vi "Init Tx - Conversion Resources.vi"(8 "error in (no error)":errorcluster, 11 "Tx Loop Data":T1) -> (0 "error out":errorcluster, 3 "Tx Loop Data out":T1)   [LabVIEW 2016, in "UDP-Custom-Device Engine.lvlib"]
uses:
  UDP-Custom-Device Engine.lvlib
  Types/Engine - Tx Loop Data.ctl
  <vilib>/NI Veristand/VeriStand Data/Byte Buffer/Byte Buffer.lvclass
  Types/Engine - General Resources.ctl
  <vilib>/NI Veristand/VeriStand Data/Typedefs/Typedefs.Data Types.ctl
  Shared/Types/Shared - Duplex Settings.ctl
  Shared/Types/Shared - Header Details.ctl
  Types/Engine - Data Conversion Config.ctl
  <vilib>/NI Veristand/VeriStand Data/Byte Buffer/Byte Buffer.Mapping.ctl
  Types/Engine - Tx Runtime Resources.ctl
  Shared/Types/Shared - Transmit Flag Options.ctl
  Types/Engine - Tx Echo Resources.ctl
  Shared/Types/Shared - Transmit Echo Options.ctl
  Types/Engine - Tx Channel Refs.ctl
  <vilib>/NI/NIVS Inline Async API/_Data Access Engine/Data Access Engine/Types/Read.DVR.ctl
  <vilib>/NI/NIVS Inline Async API/_Data Access Engine/Access Type Classes/Read/Read.lvclass
  <vilib>/NI/NIVS Inline Async API/_Data Access Engine/Data Access Engine/Types/Write.DVR.ctl
  <vilib>/NI/NIVS Inline Async API/_Data Access Engine/Access Type Classes/Write/Write.lvclass
  Types/Engine - Debug Resources.ctl
  <vilib>/NI Veristand/VeriStand Data/Byte Buffer/Byte Buffer.lvclass/Byte Buffer.ctl
  <vilib>/NI Veristand/VeriStand Data/Byte Buffer/Byte Buffer.Mapping.Create (Channel Pointer).vi
  <vilib>/NI Veristand/VeriStand Data/Utilities/Utilities.Sizeof.Array.vi
  <vilib>/NI Veristand/VeriStand Data/Memory Management/Memory Management.MoveDblBlock.Write (Double).vi
  <vilib>/NI Veristand/VeriStand Data/Byte Buffer/Byte Buffer.Write.Typed Double Array.vi
  <vilib>/NI Veristand/VeriStand Data/Utilities/Utilities.Buffer.Double.vi
  <vilib>/NI Veristand/VeriStand Data/Utilities/Utilities.Sizeof.Scalar.vi
  <vilib>/NI Veristand/VeriStand Data/Byte Buffer/Byte Buffer.Write.vi
  <vilib>/NI Veristand/VeriStand Data/Byte Buffer/Byte Buffer.Write (1D Boolean).vi
  <vilib>/NI Veristand/VeriStand Data/Type Conversion/Type Conversion.From Double.Subset.vi
  <vilib>/NI Veristand/VeriStand Data/Type Conversion/Type Conversion.From Double.Subset (1D Boolean).vi
  <vilib>/NI Veristand/VeriStand Data/Byte Buffer/Byte Buffer.Write (1D SGL).vi
  <vilib>/NI Veristand/VeriStand Data/Type Conversion/Type Conversion.From Double.Subset (1D SGL).vi
  <vilib>/NI Veristand/VeriStand Data/Byte Buffer/Byte Buffer.Write (1D DBL).vi
  <vilib>/NI Veristand/VeriStand Data/Byte Buffer/Byte Buffer.Write (1D I8).vi
  <vilib>/NI Veristand/VeriStand Data/Type Conversion/Type Conversion.From Double.Subset (1D I8).vi
  <vilib>/NI Veristand/VeriStand Data/Byte Buffer/Byte Buffer.Write (1D I16).vi
  <vilib>/NI Veristand/VeriStand Data/Type Conversion/Type Conversion.From Double.Subset (1D I16).vi
  <vilib>/NI Veristand/VeriStand Data/Byte Buffer/Byte Buffer.Write (1D I32).vi
  <vilib>/NI Veristand/VeriStand Data/Type Conversion/Type Conversion.From Double.Subset (1D I32).vi
  <vilib>/NI Veristand/VeriStand Data/Byte Buffer/Byte Buffer.Write (1D I64).vi
  <vilib>/NI Veristand/VeriStand Data/Type Conversion/Type Conversion.From Double.Subset (1D I64).vi
  <vilib>/NI Veristand/VeriStand Data/Byte Buffer/Byte Buffer.Write (1D U8).vi
  <vilib>/NI Veristand/VeriStand Data/Type Conversion/Type Conversion.From Double.Subset (1D U8).vi
  <vilib>/NI Veristand/VeriStand Data/Byte Buffer/Byte Buffer.Write (1D U16).vi
  <vilib>/NI Veristand/VeriStand Data/Type Conversion/Type Conversion.From Double.Subset (1D U16).vi
  <vilib>/NI Veristand/VeriStand Data/Byte Buffer/Byte Buffer.Write (1D U32).vi
  <vilib>/NI Veristand/VeriStand Data/Type Conversion/Type Conversion.From Double.Subset (1D U32).vi
  <vilib>/NI Veristand/VeriStand Data/Byte Buffer/Byte Buffer.Write (1D U64).vi
  <vilib>/NI Veristand/VeriStand Data/Type Conversion/Type Conversion.From Double.Subset (1D U64).vi
  <vilib>/NI Veristand/VeriStand Data/Byte Buffer/Byte Buffer.Write (String).vi
  <vilib>/NI Veristand/VeriStand Data/Type Conversion/Type Conversion.From Double.vi
  <vilib>/NI Veristand/VeriStand Data/Type Conversion/Type Conversion.From Double (1D Boolean).vi
  <vilib>/NI Veristand/VeriStand Data/Type Conversion/Type Conversion.From Double (1D SGL).vi
  <vilib>/NI Veristand/VeriStand Data/Type Conversion/Type Conversion.From Double (1D I8).vi
  <vilib>/NI Veristand/VeriStand Data/Type Conversion/Type Conversion.From Double (1D I16).vi
  <vilib>/NI Veristand/VeriStand Data/Type Conversion/Type Conversion.From Double (1D I32).vi
  <vilib>/NI Veristand/VeriStand Data/Type Conversion/Type Conversion.From Double (1D I64).vi
  <vilib>/NI Veristand/VeriStand Data/Type Conversion/Type Conversion.From Double (1D U8).vi
  <vilib>/NI Veristand/VeriStand Data/Type Conversion/Type Conversion.From Double (1D U16).vi
  <vilib>/NI Veristand/VeriStand Data/Type Conversion/Type Conversion.From Double (1D U32).vi
  <vilib>/NI Veristand/VeriStand Data/Type Conversion/Type Conversion.From Double (1D U64).vi
  <vilib>/NI Veristand/VeriStand Data/Byte Buffer/Byte Buffer.Subset.Set.vi
  <vilib>/NI Veristand/VeriStand Data/Byte Buffer/Byte Buffer.Get Buffer Pointer.vi
  <vilib>/NI Veristand/VeriStand Data/Byte Buffer/Byte Buffer.Get Buffer Size.vi
  <vilib>/NI Veristand/VeriStand Data/Memory Management/Memory Management.MoveByteBlock.Read (String).vi
  <vilib>/NI Veristand/VeriStand Data/Memory Management/Memory Management.Handle Return.vi
  <vilib>/NI Veristand/VeriStand Data/Byte Buffer/Byte Buffer.Get Byte Order.vi
  <vilib>/NI Veristand/VeriStand Data/VeriStand Data.lvlib
  <vilib>/NI/NIVS Inline Async API/_Data Access Engine/Data Access Engine/Data Access Engine.lvclass
  Shared/UDP-Custom-Device Shared.lvlib
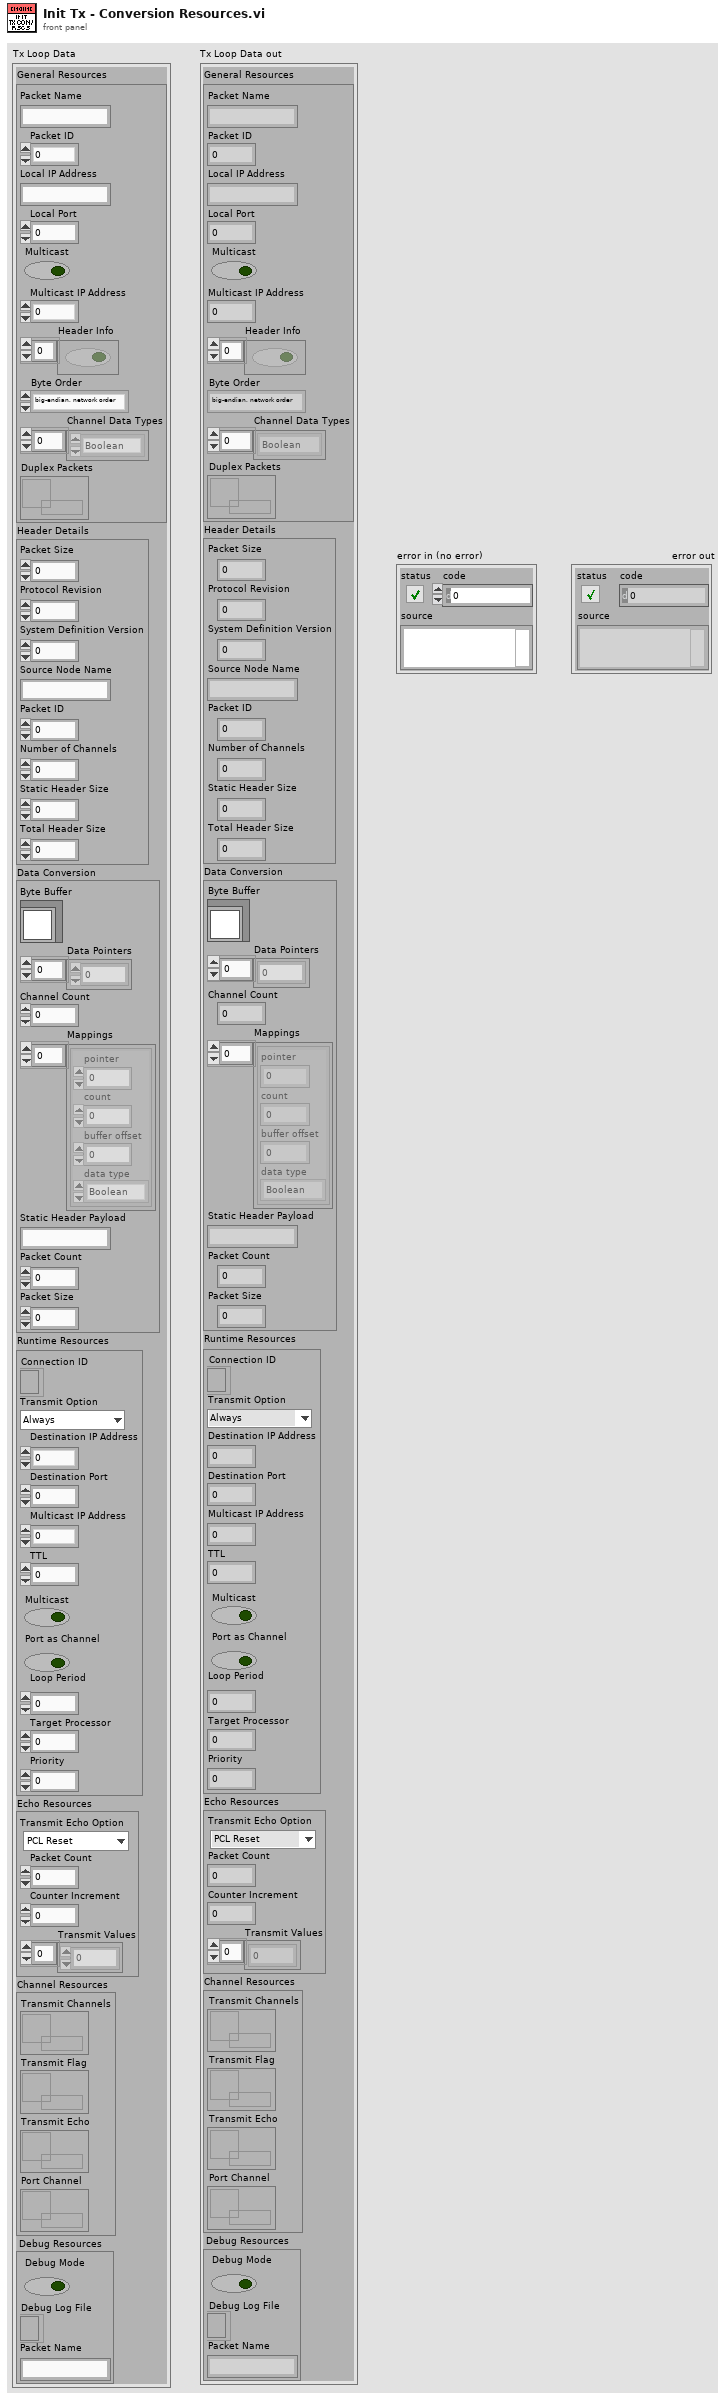
[diagram p1: front panel]
types:
  T1 = typedef "UDP-Custom-Device Engine.lvlib/Engine - Tx Loop Data.ctl" = cluster{"General Resources":T2, "Header Details":T4, "Data Conversion":T5, "Runtime Resources":T7, "Echo Resources":T9, "Channel Resources":T11, "Debug Resources":T14}
  T2 = typedef "UDP-Custom-Device Engine.lvlib/Engine - General Resources.ctl" = cluster{"Packet Name":string, "Packet ID":i32, "Local IP Address":string, "Local Port":i32, "Multicast":bool, "Multicast IP Address":u32, "Header Info":bool[], "Byte Order":enum16{"big-endian, network order", "native, host order", "little-endian"}, "Channel Data Types":T3[], "Duplex Packets":refnum<data-value>}
  T3 = typedef "VeriStand Data.lvlib/Typedefs.Data Types.ctl" = enum16{"Boolean", "Single", "Double", "I8", "I16", "I32", "I64", "U8", "U16", "U32", "U64"}
  T4 = typedef "UDP-Custom-Device Shared.lvlib/Shared - Header Details.ctl" = cluster{"Packet Size":u16, "Protocol Revision":u8, "System Definition Version":u64, "Source Node Name":string, "Packet ID":u32, "Number of Channels":u32, "Static Header Size":u16, "Total Header Size":u16}
  T5 = typedef "UDP-Custom-Device Engine.lvlib/Engine - Data Conversion Config.ctl" = cluster{"Byte Buffer":refnum<class "Byte Buffer.lvclass">, "Data Pointers":u64[], "Channel Count":i32, "Mappings":T6[], "Static Header Payload":string, "Packet Count":dbl, "Packet Size":i32}
  T6 = typedef "VeriStand Data.lvlib/Byte Buffer.lvclass/Byte Buffer.Mapping.ctl" = cluster{"pointer":u64, "count":i64, "buffer offset":u64, "data type":T3}
  T7 = typedef "UDP-Custom-Device Engine.lvlib/Engine - Tx Runtime Resources.ctl" = cluster{"Connection ID":refnum<k16>, "Transmit Option":T8, "Destination IP Address":u32, "Destination Port":u16, "Multicast IP Address":u32, "TTL":u16, "Multicast":bool, "Port as Channel":bool, "Loop Period":u32, "Target Processor":i32, "Priority":i32}
  T8 = typedef "UDP-Custom-Device Shared.lvlib/Shared - Transmit Flag Options.ctl" = enum16{"Always", "One-Shot", "Toggle"}
  T9 = typedef "UDP-Custom-Device Engine.lvlib/Engine - Tx Echo Resources.ctl" = cluster{"Transmit Echo Option":T10, "Packet Count":dbl, "Counter Increment":dbl, "Transmit Values":dbl[]}
  T10 = typedef "UDP-Custom-Device Shared.lvlib/Shared - Transmit Echo Options.ctl" = enum16{"PCL Reset", "Counter", "Mirror"}
  T11 = typedef "UDP-Custom-Device Engine.lvlib/Engine - Tx Channel Refs.ctl" = cluster{"Transmit Channels":T12, "Transmit Flag":T12, "Transmit Echo":T13, "Port Channel":T12}
  T12 = typedef "Data Access Engine.lvlib/Data Access Engine.lvclass/Read.DVR.ctl" = refnum<data-value>
  T13 = typedef "Data Access Engine.lvlib/Data Access Engine.lvclass/Write.DVR.ctl" = refnum<data-value>
  T14 = typedef "UDP-Custom-Device Engine.lvlib/Engine - Debug Resources.ctl" = cluster{"Debug Mode":bool, "Debug Log File":refnum<file>, "Packet Name":string}
  T15 = enum16{"big-endian, network order", "native, host order", "little-endian"}
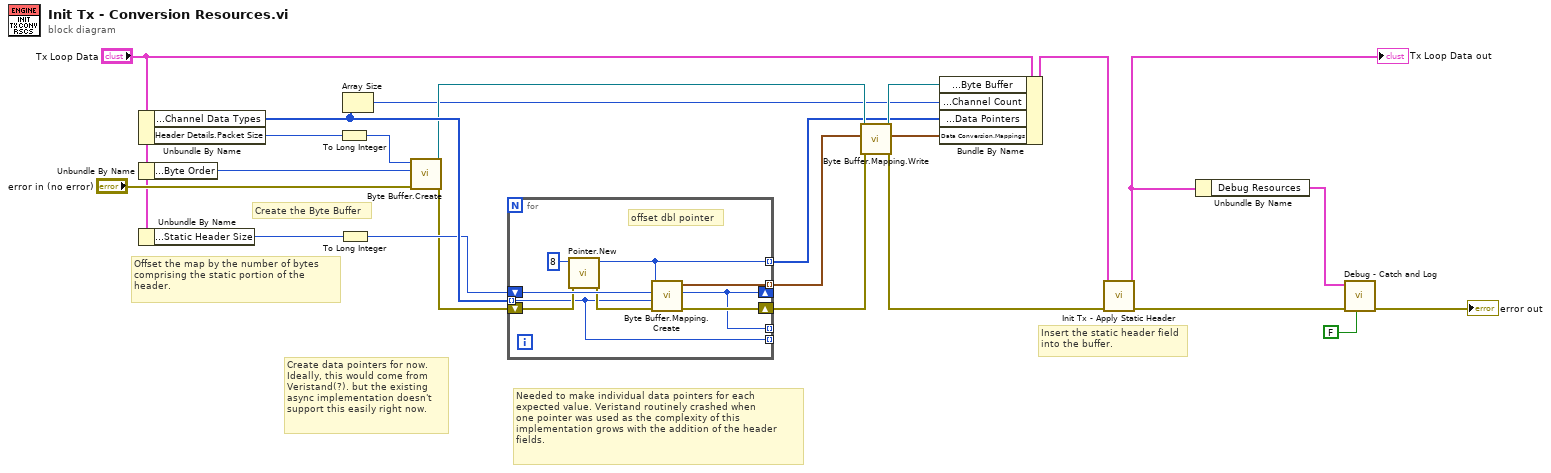
[diagram p0: block diagram]
diagram:
  # "Needed to make individual data pointers for each\nexpected value. Veristand routinely crashed when\none pointer was used as the complexity of this\nimplementation grows with the addition of the header\nfields."
  # "Insert the static header field\ninto the buffer."
  # "Offset the map by the number of bytes\ncomprising the static portion of the\nheader."
  # "Create the Byte Buffer"
  # "Create data pointers for now.\nIdeally, this would come from\nVeristand(?). but the existing\nasync implementation doesn't\nsupport this easily right now."
  n1 = Unbundle By Name("Tx Loop Data") -> ("General Resources.Channel Data Types"=w22:T3[], "Header Details.Packet Size"=w20:u16)
  n2 = Unbundle By Name("Tx Loop Data") -> ("General Resources.Byte Order"=w23:T15)
  n3 = Unbundle By Name("Tx Loop Data") -> ("Header Details.Static Header Size"=w17:u16)
  n4 = To Long Integer(number=w20) -> (32bit integer=w10:i32)
  n5 = To Long Integer(number=w17) -> (32bit integer=w9:i32)
  n6 = Array Size(array=w22) -> (size(s)=w8:i32)
  n7 = call <vilib>:"Byte Buffer.Create.vi"("error in (no error)"="error in (no error)", "byte order (big-endian)"=w23, "size"=w10) -> ("error out"=w7:errorcluster, "Byte Buffer"=w16:refnum<class "Byte Buffer.lvclass">)  [unwired: 7 in]
  n8 = for {
    tunnel: [w32] -> w13 mode=indexing
    tunnel: w22 -> [w24] mode=indexing
    shift-right: [w31] -> w12
    shift-left: w7 -> [w29]
    shift-right: [w25] -> _
    shift-left: w9 -> [w30]
    tunnel: [w26] -> w6 mode=indexing
    tunnel: [w25] -> _ mode=indexing
    tunnel: [w24] -> _ mode=indexing
    # "offset dbl pointer"
    n9 = call <vilib>:"Pointer.New.vi"("error in (no error)"=w29, "size in bytes"=8) -> ("error out"=w28:errorcluster, "pointer"=w26:u64)  [unwired: 8 in]
    n10 = call-poly <vilib>:"Byte Buffer.Mapping.Create.vi"("error in (no error)"=w28, "data type"=w24, "buffer offset"=w30, "Channel Pointer"=w26) -> ("error out"=w31:errorcluster, "new buffer offset"=w25:u64, "mapping"=w32:T6)  [unwired: 5 in]
  }
  n11 = call <vilib>:"Byte Buffer.Mapping.Write.vi"("error in (no error)"=w12, "mappings"=w13, "Byte Buffer in"=w16) -> ("error out"=w11:errorcluster, "mappings dup"=w14:T6[], "Byte Buffer out"=w15:refnum<class "Byte Buffer.lvclass">)  [unwired: 6 in]
  n12 = Bundle By Name(cluster="Tx Loop Data", "Data Conversion.Byte Buffer"=w15, "Data Conversion.Channel Count"=w8, "Data Conversion.Data Pointers"=w6, "Data Conversion.Mappings"=w14) -> (w19:T1)
  n13 = call "Init Tx - Apply Static Header.vi"("error in (no error)"=w11, "Tx Loop Data"=w19) -> ("error out"=w2:errorcluster, "Tx Loop Data out"=w3:T1)  [unwired: 8 in]
  "Tx Loop Data out" <- w3
  n14 = Unbundle By Name(w3) -> ("Debug Resources"=w4:T14)
  n15 = call "Debug - Catch and Log.vi"("Clear Error?"=FALSE, "error in (no error)"=w2, "Debug Resources"=w4) -> ("error out"=→"error out":errorcluster)  [unwired: 8 in]
